vi "CCE MGLD PMJD PF SubVI03.vi"(8 "tapa?":bool, 9 "y":sgl, 10 "x":sgl, 11 "Image 2":T1) -> (2 "Array":i32[](array[numeric]), 3 "Image":T1(plugin-control))   [LabVIEW 2020]
doc: "Ceballos Conde Emanuel Meneses Gutiérrez Luis David Pineda Méndez Job Daniel 4MV6 Sistemas de visión artificial 2022/1 \nEste vi obtiene el color de la taparrosca y etiqueta previamente detectadas utilizando el espectro de color de cada zona respectivamente"
uses:
  <vilib>/vision/Image Controls.llb/IMAQ Image.ctl
  <vilib>/vision/NI_Vision_Development_Module.lvlib
panel:
  out "max value":dbl
  in  "Color Sensitivity":u32(ring) items=["Low", "Medium", "High"]
  out "Color Spectrum":dbl[](array[numeric]) format="%.2f"
  # "Ceballos Conde Emanuel   -  Meneses Gutiérrez Luis David   -  Pineda Méndez Job Daniel 4MV6 Sistemas de visión artificial  2022/1             SubVI03"
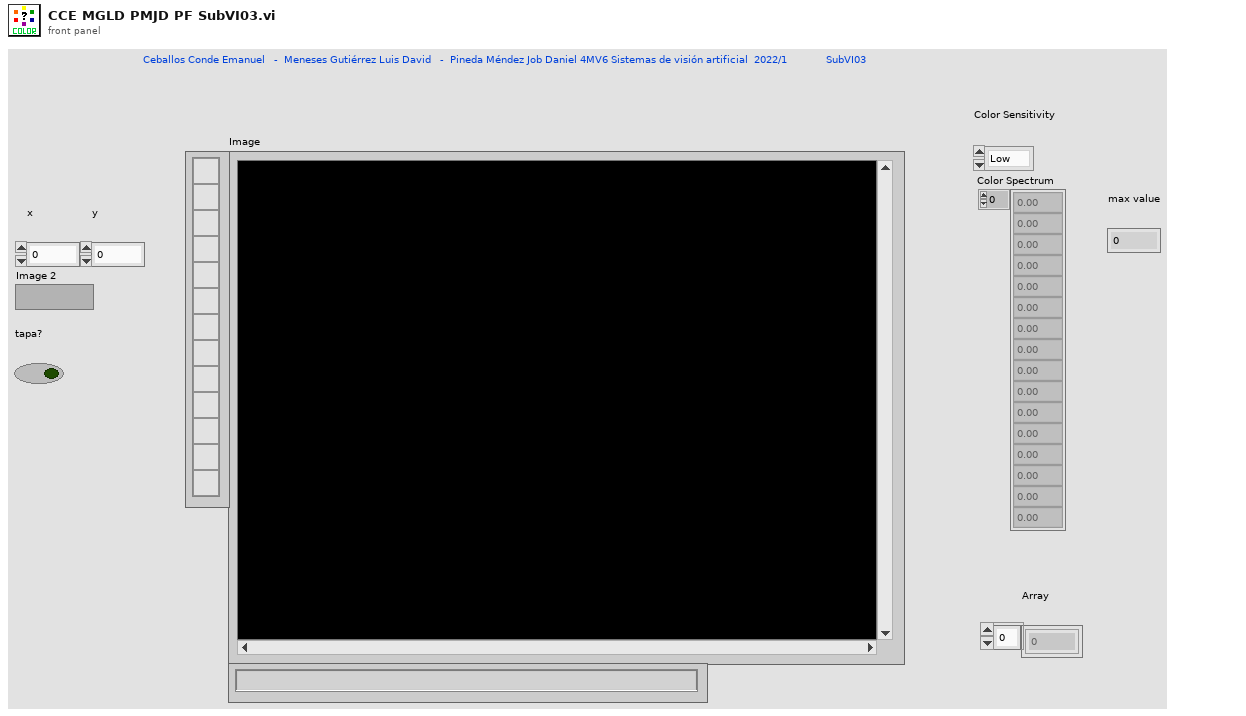
[diagram p1: front panel]
types:
  T1 = typedef "IMAQ Image.ctl" = refnum<image>
  T2 = typedef "ROI Descriptor" = cluster{"Global Rectangle":i32[], "Contours":cluster{"ID":enum32{"External", "Internal"}, "Type":u32, "Coordinates":i32[]}[]}
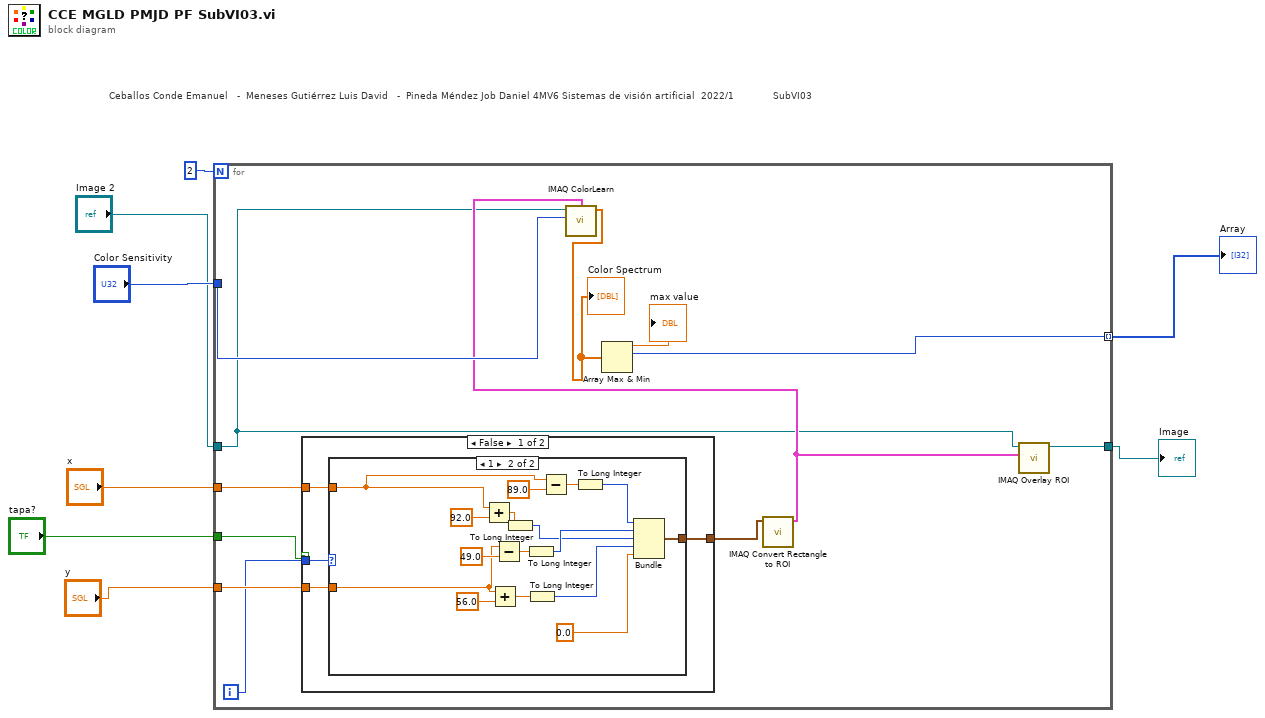
[diagram p0: block diagram]
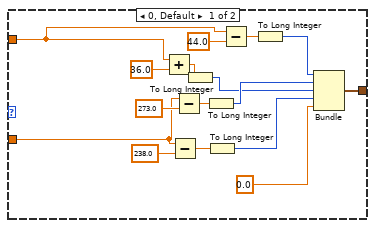
[diagram p2: hidden frame]
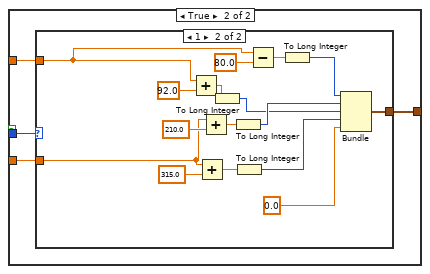
[diagram p3: hidden frame]
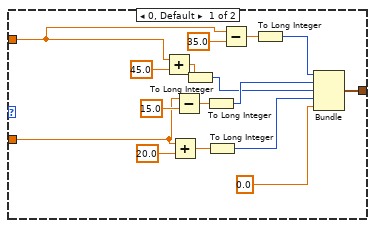
[diagram p4: hidden frame]
diagram:
  # "Ceballos Conde Emanuel   -  Meneses Gutiérrez Luis David   -  Pineda Méndez Job Daniel 4MV6 Sistemas de visión artificial  2022/1             SubVI03"
  n1 = for {
    N: 2 -> [_]
    tunnel: "Color Sensitivity" -> [w20]
    tunnel: "y" -> [w13]
    tunnel: "x" -> [w12]
    tunnel: [w10] -> w2 mode=indexing
    tunnel: "tapa?" -> [w9]
    tunnel: "Image 2" -> [w15]
    tunnel: [w14] -> w6
    i -> [w11]
    n2 = case shown="False" w9 {
      tunnel: [w24 w60] -> w17
      tunnel: w13 -> [w23 w59]
      tunnel: w12 -> [w22 w58]
      tunnel: w11 -> [w21 w57]
      frame False {
        n3 = case shown="1" w21 {
          tunnel: [w27 w43] -> w24
          tunnel: w23 -> [w26 w42]
          tunnel: w22 -> [w25 w41]
          frame 0, Default {
            n4 = Add(x=w25, y=sgl 36.0) -> (x+y=w37:sgl)
            n5 = Subtract(x=w26, y=sgl 238.0) -> (x-y=w38:sgl)
            n6 = Subtract(x=w26, y=sgl 273.0) -> (x-y=w39:sgl)
            n7 = To Long Integer(number=w37) -> (32bit integer=w29:i32)
            n8 = To Long Integer(number=w39) -> (32bit integer=w30:i32)
            n9 = To Long Integer(number=w38) -> (32bit integer=w28:i32)
            n10 = Subtract(x=w25, y=sgl 44.0) -> (x-y=w40:sgl)
            n11 = To Long Integer(number=w40) -> (32bit integer=w35:i32)
            n12 = Bundle(w35, w30, w29, w28, 0.0) -> (w27:cluster{i32, i32, i32, i32, dbl})  [unwired: 1 in]
          }
          frame 1 {
            n13 = Add(x=w41, y=sgl 92.0) -> (x+y=w53:sgl)
            n14 = Add(x=w42, y=sgl 56.0) -> (x+y=w54:sgl)
            n15 = Subtract(x=w42, y=sgl 49.0) -> (x-y=w55:sgl)
            n16 = To Long Integer(number=w53) -> (32bit integer=w45:i32)
            n17 = To Long Integer(number=w55) -> (32bit integer=w46:i32)
            n18 = To Long Integer(number=w54) -> (32bit integer=w44:i32)
            n19 = Subtract(x=w41, y=sgl 89.0) -> (x-y=w56:sgl)
            n20 = To Long Integer(number=w56) -> (32bit integer=w51:i32)
            n21 = Bundle(w51, w46, w45, w44, 0.0) -> (w43:cluster{i32, i32, i32, i32, dbl})  [unwired: 1 in]
          }
        }
      }
      frame True {
        n22 = case shown="1" w57 {
          tunnel: [w63 w79] -> w60
          tunnel: w59 -> [w62 w78]
          tunnel: w58 -> [w61 w77]
          frame 0, Default {
            n23 = Add(x=w61, y=sgl 45.0) -> (x+y=w73:sgl)
            n24 = Add(x=w62, y=sgl 20.0) -> (x+y=w74:sgl)
            n25 = Subtract(x=w62, y=sgl 15.0) -> (x-y=w75:sgl)
            n26 = To Long Integer(number=w73) -> (32bit integer=w65:i32)
            n27 = To Long Integer(number=w75) -> (32bit integer=w66:i32)
            n28 = To Long Integer(number=w74) -> (32bit integer=w64:i32)
            n29 = Subtract(x=w61, y=sgl 35.0) -> (x-y=w76:sgl)
            n30 = To Long Integer(number=w76) -> (32bit integer=w71:i32)
            n31 = Bundle(w71, w66, w65, w64, 0.0) -> (w63:cluster{i32, i32, i32, i32, dbl})  [unwired: 1 in]
          }
          frame 1 {
            n32 = Add(x=w77, y=sgl 92.0) -> (x+y=w89:sgl)
            n33 = Add(x=w78, y=sgl 315.0) -> (x+y=w90:sgl)
            n34 = Add(x=w78, y=sgl 210.0) -> (x+y=w91:sgl)
            n35 = To Long Integer(number=w89) -> (32bit integer=w81:i32)
            n36 = To Long Integer(number=w91) -> (32bit integer=w82:i32)
            n37 = To Long Integer(number=w90) -> (32bit integer=w80:i32)
            n38 = Subtract(x=w77, y=sgl 80.0) -> (x-y=w92:sgl)
            n39 = To Long Integer(number=w92) -> (32bit integer=w87:i32)
            n40 = Bundle(w87, w82, w81, w80, 0.0) -> (w79:cluster{i32, i32, i32, i32, dbl})  [unwired: 1 in]
          }
        }
      }
    }
    n41 = call "IMAQ Convert Rectangle to ROI"("Rectangle"=w17) -> ("ROI Descriptor"=w16:T2)  [unwired: 8 in, 1 out]
    n42 = call "IMAQ ColorLearn"("ROI Descriptor"=w16, "Image"=w15, "Color Sensitivity"=w20) -> ("Color Spectrum"=w19:dbl[])  [unwired: 5 in, 1 out]
    "Color Spectrum" <- w19
    n43 = Array Max & Min(array=w19) -> (max value=→"max value":dbl, max index (indices)=w10:i32)  [unwired: 2 out]
    n44 = call "IMAQ Overlay ROI"("ROI Descriptor"=w16, "Image"=w15) -> ("Image Out"=w14:T1)  [unwired: 8 in, 1 out]
  }
  "Image" <- w6
  "Array" <- w2
